vi "))Channel.vi"(7 "This VI":refnum<vi>, 8 "Remove Queue":refnum<queue>, 9 "New Queue Depth":i32, 10 "channelOp":T3=enum."Close", 11 "channel in":T2) -> (1 "New Queue":refnum<queue>, 2 "Channel Data":T1, 3 "channel out":T2, 5 "This VI out":refnum<vi>)   [LabVIEW 2020, in "Flex.lvlib"]
uses:
  Flex.lvlib
  ChannelOp.ctl
  ))Channel.ctl
  Element.ctl
  Channel Data.ctl
  Element Info.ctl
  Instantiate.vi
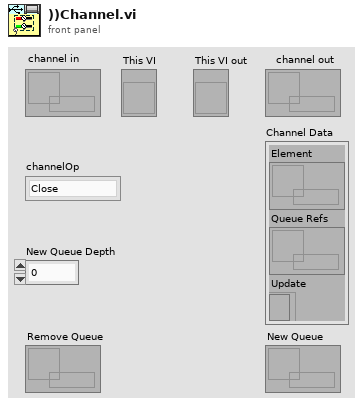
[diagram p1: front panel]
types:
  T1 = typedef "Flex.lvlib/Channel Data.ctl" = cluster{"Element":refnum<data-value>, "Queue Refs":refnum<data-value>, "Update":refnum<k4>}
  T2 = typedef "Flex.lvlib/))Channel.ctl" = refnum<queue>
  T3 = typedef "Flex.lvlib/ChannelOp.ctl" = enum16{"Get Refs", "Init", "Close", "Probe", "New Queue", "Remove Queue"}
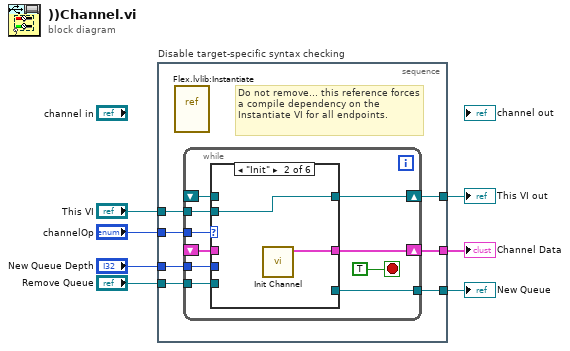
[diagram p0: block diagram]
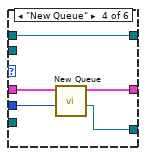
[diagram p4: hidden frame]
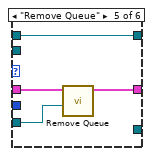
[diagram p5: hidden frame]
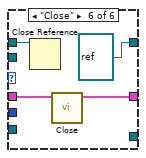
[diagram p6: hidden frame]
diagram:
  n1 = stacked-sequence "Disable target-specific syntax checking" {
    tunnel: "channelOp" -> [w14]
    tunnel: "This VI" -> [w13]
    tunnel: [w12] -> w5
    tunnel: "New Queue Depth" -> [w11]
    tunnel: [w10] -> w3
    tunnel: [w9] -> w2
    tunnel: "Remove Queue" -> [w8]
    frame #0 {
      # "Do not remove... this reference forces a compile dependency on the Instantiate VI for all endpoints."
      n2 = vi-ref "Flex.lvlib:Instantiate.vi"() -> ()  [unwired: 1 out]
      n3 = while {
        tunnel: w14 -> [w22]
        shift-right: [w18] -> w9
        shift-left: _ -> [w24]
        shift-right: [w19] -> w12
        shift-left: _ -> [w20]
        tunnel: w13 -> [w21]
        tunnel: w11 -> [w17]
        tunnel: [w16] -> w10
        tunnel: w8 -> [w15]
        stop <- TRUE stop-if-true
        n4 = case shown="\"Init\"" w22 {
          tunnel: [w25 w27 w29 w33 w37 w40] -> w18
          tunnel: w24 -> [w25 _ w29 w34 w38 w41]
          tunnel: w21 -> [_ w28 _ _ _ _]
          tunnel: [w26 w28 w30 w35 w39 refnum<vi> refnum ("This VI")] -> w19
          tunnel: w20 -> [w26 _ w30 w35 w39 w42]
          tunnel: w17 -> [_ _ _ w32 _ _]
          tunnel: [_ _ _ w31 _ _] -> w16
          tunnel: w15 -> [_ _ _ _ w36 _]
          frame "Get Refs" {
          }
          frame "Init" {
            n5 = call "Init Channel.vi"() -> ("Channel Data"=w27:T1)  [unwired: 11 in]
          }
          frame "Probe" {
          }
          frame "New Queue" {
            n6 = call "New Queue.vi"("Depth"=w32, "Channel Data In"=w34) -> ("Queue"=w31:refnum<queue>, "Channel Data"=w33:T1)  [unwired: 8 in]
          }
          frame "Remove Queue" {
            n7 = call "Remove Queue.vi"("Queue"=w36, "Channel Data In"=w38) -> ("Channel Data"=w37:T1)  [unwired: 9 in]
          }
          frame "Close" {
            n8 = Close Reference(reference=w42) -> ()  [unwired: 1 in, 1 out]
            n9 = call "Close.vi"("Channel Data In"=w41) -> ("Channel Data"=w40:T1)  [unwired: 10 in]
          }
        }
      }
    }
  }
  "This VI out" <- w5
  "New Queue" <- w3
  "Channel Data" <- w2
